vi "SPI Set Clock Divider.vi"(0 "Arduino Resource":T1={"VISA resource"="", "Board Type"=enum."Arduino Uno", "Connection Type"=enum."USB / Serial", "Bytes Per Packet (15)"=15}, 7 "SPI Clock Divider":T3, 11 "error in":errorcluster) -> (4 "Arduino Resource":T1={"VISA resource"="", "Board Type"=enum."Arduino Uno", "Connection Type"=enum."USB / Serial", "Bytes Per Packet (15)"=15}, 15 "error out":errorcluster)   [LabVIEW 2011, in "LabVIEW Interface for ChipKit.lvlib"]
doc: "Set the SPI clock divider.s"
uses:
  <vilib>/LabVIEW Interface for ChipKit/LabVIEW Interface for ChipKit.lvlib
  <vilib>/LabVIEW Interface for ChipKit/Private/Type Defs/SPI Clock Divider.ctl
  <vilib>/LabVIEW Interface for ChipKit/Private/Type Defs/Chipkit Resource.ctl
  <vilib>/LabVIEW Interface for ChipKit/Private/Type Defs/Board Type.ctl
  <vilib>/LabVIEW Interface for ChipKit/Private/Type Defs/Command.ctl
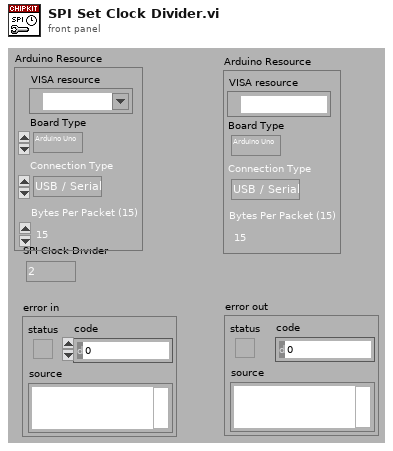
[diagram p1: front panel]
types:
  T1 = typedef "LabVIEW Interface for ChipKit.lvlib/Chipkit Resource.ctl" = cluster{"VISA resource":refnum<visa-resource-name>, "Board Type":T2, "Connection Type":enum8{"USB / Serial"}, "Bytes Per Packet (15)":u8}
  T2 = typedef "LabVIEW Interface for ChipKit.lvlib/Board Type.ctl" = enum16{"Arduino Uno", "Dimuelanove w/Atmega 328", "Mega 2560", "Chipkit Uno32", "Chipkit Max32"}
  T3 = typedef "LabVIEW Interface for ChipKit.lvlib/SPI Clock Divider.ctl" = enum8{"2", "4", "8", "16", "32", "64", "128"}
  T4 = typedef "LabVIEW Interface for ChipKit.lvlib/Command.ctl" = enum8{"setArduinoMode", "flushSerial", "setPinMode", "digitalWritePin", "digitalWritePort", "tone", "digitalReadPin", "digitalReadPort", "analogReadPin", "analogReadPort", "pwmWritePin", "pwmWritePort", "sevenSegment_Configure", "sevenSegment_Write", "I2C Init", "I2C Write", "I2C Read", "SPI Init", "SPI Set Bit Order", "SPI Set Clock Divider", "SPI Set Data Mode", "SPI Send / Receive", "SPI Close", "Servo Set Num Servos", "Servo Config Servo", "Servo Write Angle", "Servo Read Angle", "Servo Write Pulse Width", "Servo Read Pulse Width", "Servo Detach", "LCD Init", "LCD Set Size", "LCD Set Cursor Mode", "LCD Clear", "LCD Set Cursor Position", "LCD Print", "LCD Display Power", "LCD Scroll Display", "LCD Autoscroll", "LCD Print Direction", "LCD Create Custom Char", "LCD Print Custom Char", "contAcqOn", "contAcqOff", "getFirmwareVersion", "FiniteSampleStart"}
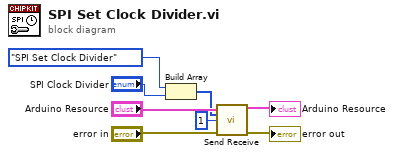
[diagram p0: block diagram]
diagram:
  n1 = Build Array(Command."SPI Set Clock Divider" ("Command"), "SPI Clock Divider") -> (w2:u8[])
  n2 = call <vilib>:"Send Receive.vi"("Arduino Resource"="Arduino Resource", "Data"=w2, "Bytes To Read (0)"=u32 1, "error in"="error in") -> ("Arduino Resource"=→"Arduino Resource":T1, "error out"=→"error out":errorcluster)  [unwired: 9 in, 1 out]
